vi "Memory.Pointer.Read.All.In Place.Unsafe (1D U8).vi"(8 "error in (no error)":errorcluster, 10 "buffer in":u8[](array[numeric]) format="%02x", 11 "Pointer in":refnum<class "Memory.Pointer.lvclass">) -> (0 "error out":errorcluster, 2 "buffer out":u8[](array[numeric]) format="%02x", 3 "Pointer out":refnum<class "Memory.Pointer.lvclass">)   [LabVIEW 2016, in "LabVIEW Memory Manager.lvlib" / "Memory.Pointer.lvclass"]
uses:
  Memory.Pointer.lvclass
  Memory.Pointer.lvclass/Memory.Pointer.ctl
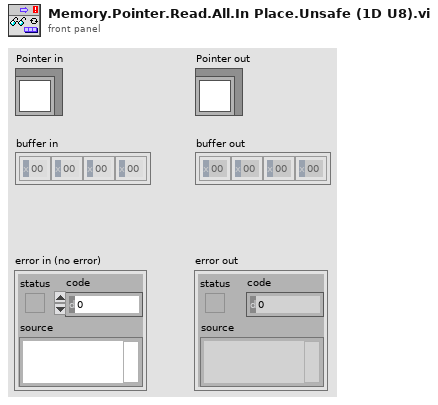
[diagram p1: front panel]
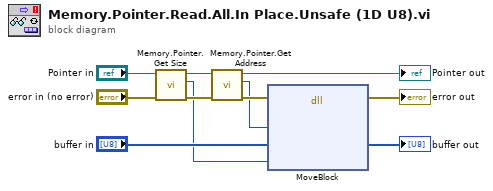
[diagram p0: block diagram]
diagram:
  n1 = call "Memory.Pointer.Get Size.vi"("error in (no error)"="error in (no error)", "Pointer in"="Pointer in") -> ("error out"=w11:errorcluster, "size"=w1:i64, "Pointer out"=w10:refnum<class "Memory.Pointer.lvclass">)  [unwired: 7 in]
  n2 = call "Memory.Pointer.Get Address.vi"("error in (no error)"=w11, "Pointer in"=w10) -> ("error out"=w9:errorcluster, "address"=w8:u64, "Pointer out"=→"Pointer out":refnum<class "Memory.Pointer.lvclass">)  [unwired: 7 in]
  n3 = dll-call lib="LabVIEW" fn="MoveBlock"(error in=w9, "src pointer"=w8, "dst pointer"="buffer in", "size"=w1) -> (error out=→"error out":errorcluster, "dst pointer"=→"buffer out":u8[])  [unwired: 5 in, 1 out]
